vi "ADC_config_fastsweep.vi"(0 "Inst_parameter":T1, 1 "Fast sequence size":u32, 2 "fast sequence divider":u32, 3 "Ramp?":bool=TRUE) -> (5 "Inst_parameter out":T1)   [LabVIEW 2013]
uses:
  <vilib>/DAQmx/create/channels.llb/DAQmx Create Channel (AI-Voltage-Basic).vi
  <vilib>/DAQmx/configure/timing.llb/DAQmx Timing (Sample Clock).vi
  <vilib>/DAQmx/create/channels.llb/DAQmx Create Channel (CO-Pulse Generation-Frequency).vi
  <vilib>/DAQmx/configure/timing.llb/DAQmx Timing (Implicit).vi
  <vilib>/DAQmx/configure/trigger.llb/DAQmx Start Trigger (Digital Edge).vi
  <resource>/objmgr/daqmx.rc
panel:
  out "error out":errorcluster
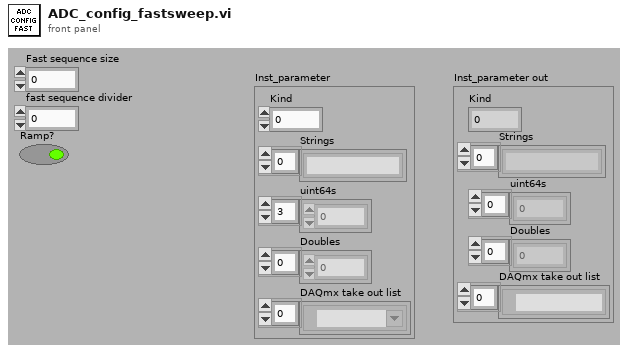
[diagram p1: front panel]
types:
  T1 = cluster{"Kind":u16, "Strings":string[], "uint64s":u64[], "Doubles":dbl[], "DAQmx take out list":refnum<k21>[]}
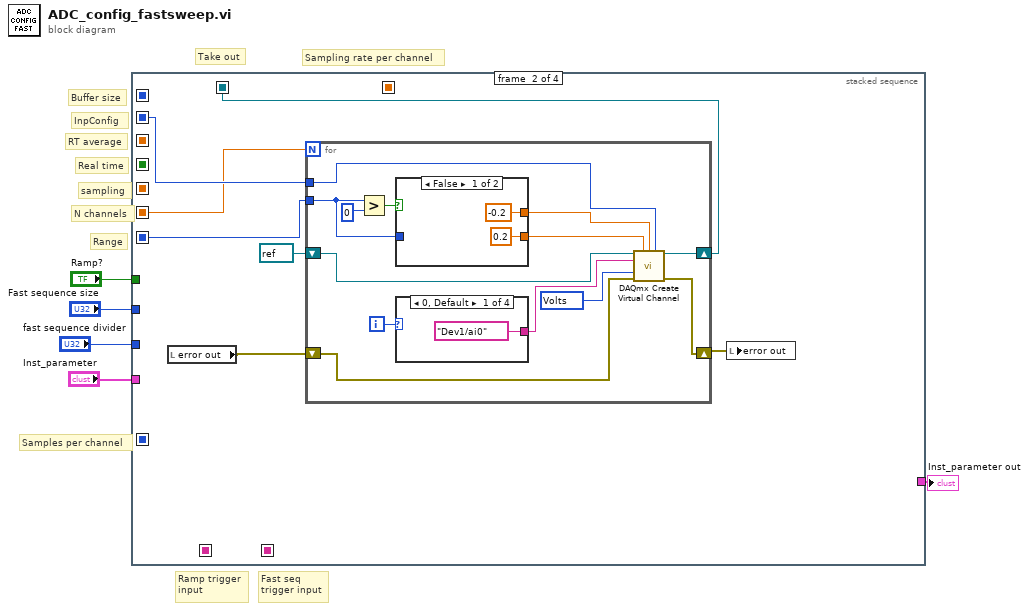
[diagram p0: block diagram]
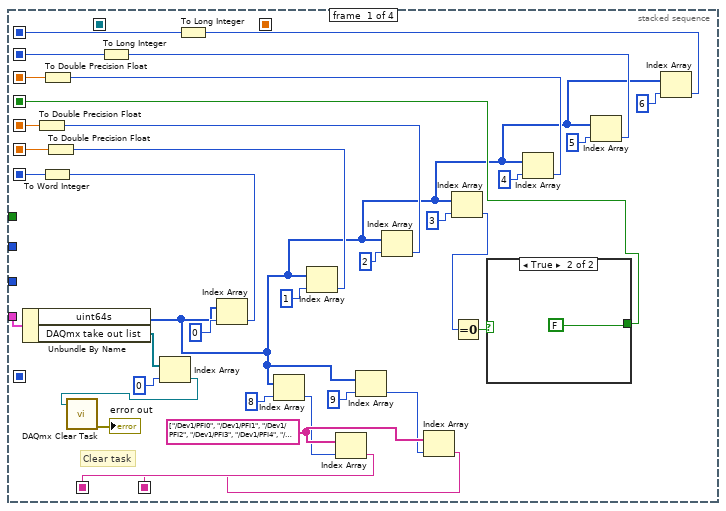
[diagram p2: hidden frame]
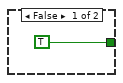
[diagram p3: hidden frame]
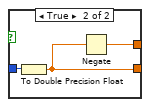
[diagram p4: hidden frame]
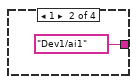
[diagram p5: hidden frame]
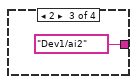
[diagram p6: hidden frame]
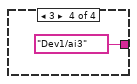
[diagram p7: hidden frame]
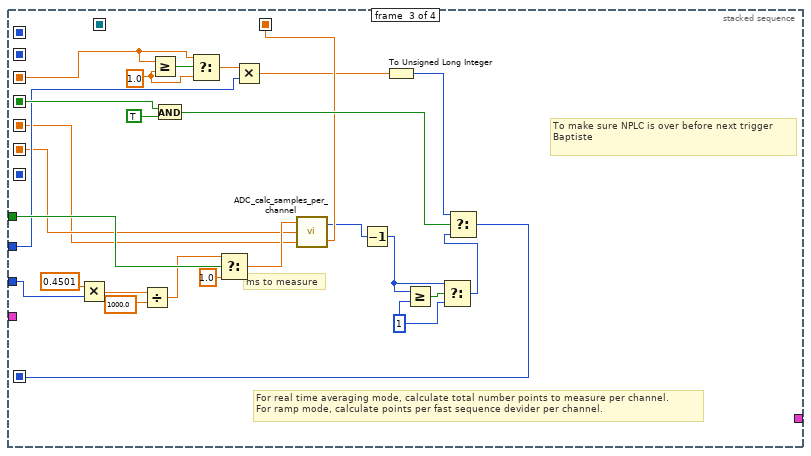
[diagram p8: hidden frame]
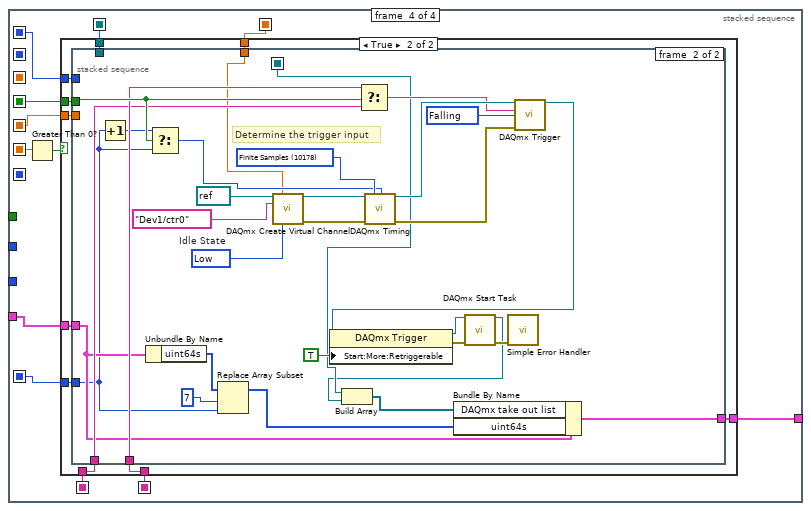
[diagram p9: hidden frame]
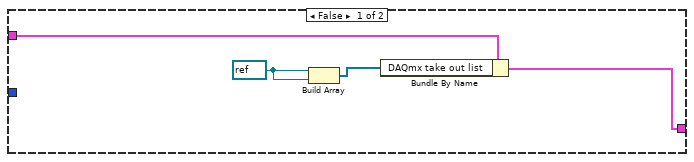
[diagram p10: hidden frame]
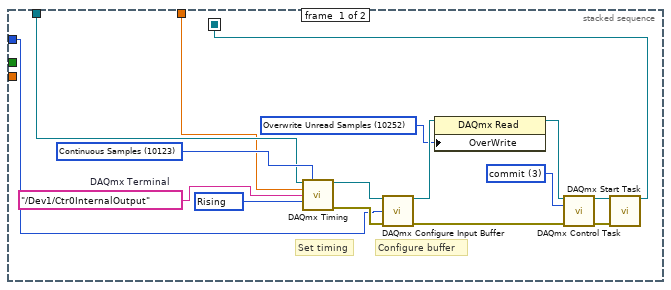
[diagram p11: hidden frame]
diagram:
  # "Fast seq \ntrigger input"
  # "Ramp trigger\ninput"
  # "Take out"
  # "Sampling rate per channel"
  # "Samples per channel"
  # "Buffer size"
  # "InpConfig"
  # "RT average"
  # "Real time"
  # "sampling"
  # "N channels"
  # "Range"
  n1 = stacked-sequence {
    seq-local: [w25 _ _ _] -> [_ _ _ w106]
    seq-local: [w20 _ _ _] -> [_ w48 _ _]
    seq-local: [w23 _ _ _] -> [_ _ w75 _]
    seq-local: [w17 _ _ _] -> [_ _ w98 w105]
    seq-local: [w22 _ _ _] -> [_ _ w83 w99]
    seq-local: [w24 _ _ _] -> [_ w44 w84 w110]
    seq-local: [w21 _ _ _] -> [_ w47 _ _]
    seq-local: [_ _ w78 _] -> [_ _ _ w104]
    seq-local: [_ _ w86 _] -> [_ _ _ w108]
    seq-local: [_ w43 _ _] -> [_ _ _ w107]
    seq-local: [w7 _ _ _] -> [_ _ _ w102]
    seq-local: [w6 _ _ _] -> [_ _ _ w103]
    tunnel: "Inst_parameter" -> [w39 _ _ w101]
    tunnel: "Fast sequence size" -> [_ _ w87 _]
    tunnel: "fast sequence divider" -> [_ _ w93 _]
    tunnel: "Ramp?" -> [_ _ w97 _]
    tunnel: [_ _ _ w100] -> w2
    frame #0 {
      w10 = tag[] ["/Dev1/PFI0", "/Dev1/PFI1", "/Dev1/PFI2", "/Dev1/PFI3", "/Dev1/PFI4", "/Dev1/PFI5", "/Dev1/PFI6", "/Dev1/PFI7", "/Dev1/PFI8", "/Dev1/PFI9", "/Dev1/PFI10", "/Dev1/PFI11", "/Dev1/PFI12"]
      # "Clear task"
      n2 = Unbundle By Name(w39) -> ("uint64s"=w13:u64[], "DAQmx take out list"=w15:refnum<k21>[])
      n3 = Index Array(array=w15, index=0) -> (element=w14:refnum<k21>)
      n4 = call <vilib>:"DAQmx Clear Task.vi"("task in"=w14) -> ("error out"=→"error out":errorcluster)  [unwired: 14 in]
      n5 = Index Array(array=w13, index=0) -> (element=w26:u64)
      n6 = To Word Integer(number=w26) -> (16bit integer=w21:i16)
      n7 = Index Array(array=w13, index=8) -> (element=w9:u64)
      n8 = Index Array(array=w13, index=1) -> (element=w27:u64)
      n9 = To Double Precision Float(number=w27) -> (double precision float=w24:dbl)
      n10 = Index Array(array=w10, index=w9) -> (element=w7:tag)
      n11 = Index Array(array=w13, index=9) -> (element=w8:u64)
      n12 = Index Array(array=w13, index=2) -> (element=w28:u64)
      n13 = To Double Precision Float(number=w28) -> (double precision float=w22:dbl)
      n14 = Index Array(array=w10, index=w8) -> (element=w6:tag)
      n15 = Index Array(array=w13, index=3) -> (element=w18:u64)
      n16 = Equal To 0?(x=w18) -> (x = 0?=w19:bool)
      n17 = case shown="True" w19 {
        tunnel: [TRUE FALSE] -> w17
        frame False {
        }
        frame True {
        }
      }
      n18 = Index Array(array=w13, index=4) -> (element=w29:u64)
      n19 = To Double Precision Float(number=w29) -> (double precision float=w23:dbl)
      n20 = Index Array(array=w13, index=5) -> (element=w30:u64)
      n21 = To Long Integer(number=w30) -> (32bit integer=w20:i32)
      n22 = Index Array(array=w13, index=6) -> (element=w31:u64)
      n23 = To Long Integer(number=w31) -> (32bit integer=w25:i32)
    }
    frame #1 {
      n24 = local read "error out"() -> (w46:errorcluster)
      n25 = for {
        N: w44 -> [_]
        shift-right: [w62] -> w43
        shift-left: refnum<k21> refnum ("task out") -> [w61]
        shift-right: [w58] -> w45
        shift-left: w46 -> [w57]
        tunnel: w47 -> [w54]
        tunnel: w48 -> [w50]
        i -> [w51]
        w59 = 10348 items=["Volts"=10348, "From Custom Scale"=10065] ("units")
        n26 = Greater?(x=w54, y=i16 0) -> (0:w55:bool)
        n27 = case shown="False" w55 {
          tunnel: w54 -> [_ w67]
          tunnel: [-0.2 w65] -> w56
          tunnel: [0.2 w66] -> w52
          frame False {
          }
          frame True {
            n28 = To Double Precision Float(number=w67) -> (double precision float=w66:dbl)
            n29 = Negate(x=w66) -> (-x=w65:dbl)
          }
        }
        n30 = case shown="0, Default" w51 {
          tunnel: [tag "Dev1/ai0" ("physical channels") tag "Dev1/ai1" ("physical channels") tag "Dev1/ai2" ("physical channels") tag "Dev1/ai3" ("physical channels")] -> w60
          frame 0, Default {
          }
          frame 1 {
          }
          frame 2 {
          }
          frame 3 {
          }
        }
        n31 = call-poly <vilib>:"DAQmx Create Virtual Channel.vi"("task in"=w61, "maximum value"=w52, "minimum value"=w56, "input terminal configuration"=w50, "physical channels"=w60, "units"=w59, "error in"=w57) -> ("task out"=w62:refnum<k21>, "error out"=w58:errorcluster)  [unwired: 2 in, 5 out]
      }
      n32 = local write "error out"(w45) -> ()
    }
    frame #2 {
      w81 = 1
      w77 = 1.0 ("t")
      # "To make sure NPLC is over before next trigger\nBaptiste"
      # "For real time averaging mode, calculate total number points to measure per channel.\nFor ramp mode, calculate points per fast sequence devider per channel."
      # "ms to measure"
      n33 = Multiply(x=0.4501, y=w93) -> (x*y=w95:dbl)
      n34 = Divide(x=w95, y=1000.0) -> (x/y=w92:dbl)
      n35 = Greater Or Equal?(x=w75, y=w77) -> (x >= y?=w76:bool)
      n36 = And(x=w98, y=TRUE) -> (x .and. y?=w89:bool)
      n37 = Select(t=w75, s=w76, f=w77) -> (s? t:f=w88:dbl)
      n38 = Select(t=w92, s=w97, f=1.0) -> (s? t:f=w85:dbl)
      n39 = Multiply(x=w88, y=w87) -> (x*y=w80:dbl)
      n40 = call "ADC_calc_samples_per_channel.vi"("Samplingrate"=w83, "Nchannel"=w84, "time per point (ms)"=w85) -> ("effective samplingrate"=w86:dbl, "samples to read"=w73:u32)
      n41 = Decrement(x=w73) -> (x-1=w74:u32)
      n42 = To Unsigned Long Integer(number=w80) -> (unsigned 32bit integer=w79:u32)
      n43 = Greater Or Equal?(x=w74, y=w81) -> (x >= y?=w82:bool)
      n44 = Select(t=w74, s=w82, f=w81) -> (s? t:f=w90:u32)
      n45 = Select(t=w79, s=w89, f=w90) -> (s? t:f=w78:u32)
    }
    frame #3 {
      n46 = Greater Than 0?(x=w110) -> (x > 0?=w109:bool)
      n47 = case shown="True" w109 {
        tunnel: w108 -> [_ w124]
        tunnel: w107 -> [_ w123]
        tunnel: w106 -> [_ w122]
        tunnel: w105 -> [_ w121]
        tunnel: w104 -> [_ w120]
        tunnel: w103 -> [_ w119]
        tunnel: w102 -> [_ w118]
        tunnel: w101 -> [w114 w117]
        tunnel: [w111 w116] -> w100
        tunnel: w99 -> [_ w115]
        frame False {
          w113 = refnum<k21> refnum ("task out")
          n48 = Build Array(w113, w113) -> (w112:refnum<k21>[])
          n49 = Bundle By Name(cluster=w114, "DAQmx take out list"=w112) -> (w111:T1)
        }
        frame True {
          n50 = stacked-sequence {
            seq-local: [w126 _] -> [_ w153]
            tunnel: w124 -> [w125 w142]
            tunnel: w123 -> [w128 _]
            tunnel: w122 -> [w127 _]
            tunnel: w121 -> [_ w155]
            tunnel: w120 -> [_ w141]
            tunnel: w119 -> [_ w151]
            tunnel: w118 -> [_ w150]
            tunnel: w117 -> [_ w149]
            tunnel: [_ w144] -> w116
            tunnel: w115 -> [_ _]
            frame #0 {
              w129 = 10252 items=["Overwrite Unread Samples"=10252, "Do Not Overwrite Unread Samples"=10159] ("OverWrite")
              w131 = 3 items=["verify"=2, "reserve"=4, "commit"=3, "unreserve"=5, "abort"=6] ("action")
              w138 = tag "/Dev1/Ctr0InternalOutput"  # DAQmx Terminal
              w139 = 10280 items=["Rising"=10280, "Falling"=10171] ("active edge")
              w140 = 10123 items=["Finite Samples"=10178, "Continuous Samples"=10123, "Hardware Timed Single Point"=12522] ("sample mode")
              # "Set timing"
              # "Configure buffer"
              n51 = call-poly <vilib>:"DAQmx Timing.vi"("task/channels in"=w128, "sample mode"=w140, "rate"=w125, "source"=w138, "active edge"=w139) -> ("task out"=w137:refnum<k21>, "error out"=w136:errorcluster)  [unwired: 9 in]
              n52 = call <vilib>:"DAQmx Configure Input Buffer.vi"("task/channels in"=w137, "buffer size (in samples per channel)"=w127, "error in"=w136) -> ("task out"=w135:refnum<k21>, "error out"=w133:errorcluster)  [unwired: 11 out]
              n53 = property class="DAQmx Read"(reference=w135, "OverWrite"=w129) -> (reference out=w130:refnum<k21>)  [unwired: 1 in, 1 out]
              n54 = call <vilib>:"DAQmx Control Task.vi"("task/channels in"=w130, "action"=w131, "error in"=w133) -> ("task out"=w134:refnum<k21>, "error out"=w132:errorcluster)  [unwired: 11 in]
              n55 = call <vilib>:"DAQmx Start Task.vi"("task/channels in"=w134, "error in"=w132) -> ("task out"=w126:refnum<k21>)  [unwired: 12 in, 1 out]
            }
            frame #1 {
              w164 = 10171 items=["Rising"=10280, "Falling"=10171] ("Trigger Edge")
              w167 = 10214 items=["High"=10192, "Low"=10214]  # Idle State
              w168 = 10178 items=["Finite Samples"=10178, "Continuous Samples"=10123] ("sample mode")
              # "Determine the trigger input"
              n56 = Increment(x=w141) -> (x+1=w143:u32)
              n57 = Unbundle By Name(w149) -> ("uint64s"=w147:u64[])
              n58 = Select(t=w143, s=w155, f=w141) -> (s? t:f=w154:u32)
              n59 = Replace Array Subset(array=w147, new element=w141, index=7) -> (w145:u64[])
              n60 = call-poly <vilib>:"DAQmx Create Virtual Channel.vi"("task in"=refnum<k21> refnum, "frequency"=w142, "counter"=tag "Dev1/ctr0", "idle state"=w167) -> ("task out"=w169:refnum<k21>, "error out"=w170:errorcluster)  [unwired: 5 in, 5 out]
              n61 = Select(t=w151, s=w155, f=w150) -> (s? t:f=w162:tag)
              n62 = call-poly <vilib>:"DAQmx Timing.vi"("task/channels in"=w169, "sample mode"=w168, "samples per channel"=w154, "error in"=w170) -> ("task out"=w166:refnum<k21>, "error out"=w165:errorcluster)  [unwired: 2 in, 8 out]
              n63 = call-poly <vilib>:"DAQmx Trigger.vi"("task/channels in"=w166, "source"=w162, "edge"=w164, "error in"=w165) -> ("task out"=w157:refnum<k21>)  [unwired: 11 out]
              n64 = property class="DAQmx Trigger"(reference=w157, "Start:More:Retriggerable"=TRUE) -> (reference out=w156:refnum<k21>, error out=w159:errorcluster)  [unwired: 1 in]
              n65 = call <vilib>:"DAQmx Start Task.vi"("task/channels in"=w156, "error in"=w159) -> ("task out"=w152:refnum<k21>, "error out"=w158:errorcluster)  [unwired: 12 out]
              n66 = Build Array(w153, w152) -> (w148:refnum<k21>[])
              n67 = Bundle By Name(cluster=w149, "DAQmx take out list"=w148, "uint64s"=w145) -> (w144:T1)
              n68 = call <vilib>:"Simple Error Handler.vi"("error in (no error)"=w158) -> ()  [unwired: 4 in, 5 out]
            }
          }
        }
      }
    }
  }
  "Inst_parameter out" <- w2
